vi "SO55 Initialize.vi"(1 "error in":errorcluster) -> (0 "error out":errorcluster, 2 "Settings Out":T1)   [LabVIEW 2012]
uses:
  SO55 Settings Cluster.ctl
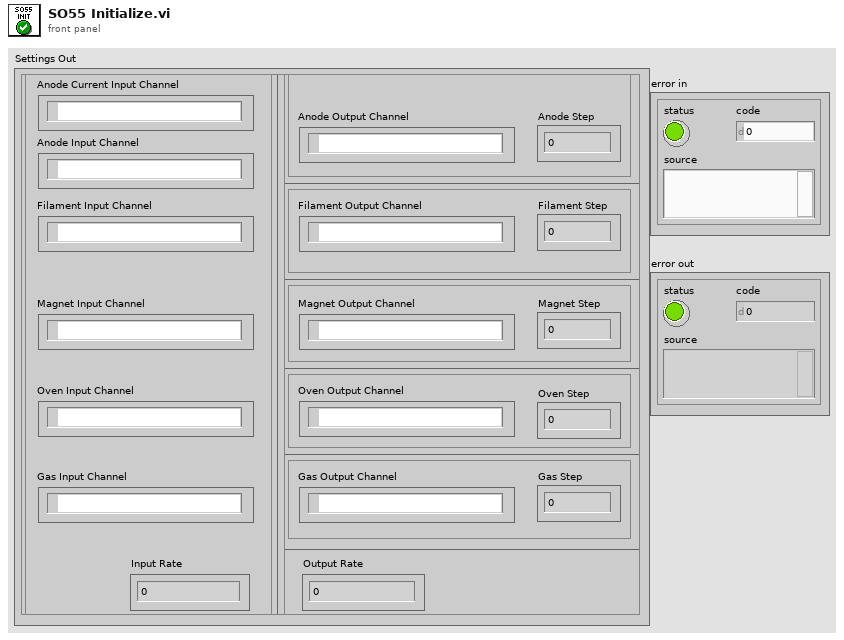
[diagram p1: front panel]
types:
  T1 = typedef "SO55 Settings Cluster.ctl" = cluster{"Input":cluster{"Anode Input Channel":tag, "Filament Input Channel":tag, "Magnet Input Channel":tag, "Oven Input Channel":tag, "Gas Input Channel":tag, "Input Rate":dbl, "Anode Current Input Channel":tag}, "Output":cluster{"Anode":cluster{"Anode Output Channel":tag, "Anode Step":dbl}, "Filament":cluster{"Filament Output Channel":tag, "Filament Step":dbl}, "Magnet":cluster{"Magnet Output Channel":tag, "Magnet Step":dbl}, "Oven":cluster{"Oven Output Channel":tag, "Oven Step":dbl}, "Gas":cluster{"Gas Output Channel":tag, "Gas Step":dbl}, "Output Rate":dbl}}
  T2 = enum16{"open", "replace", "create", "open or create", "replace or create", "replace or create with confirmation"}
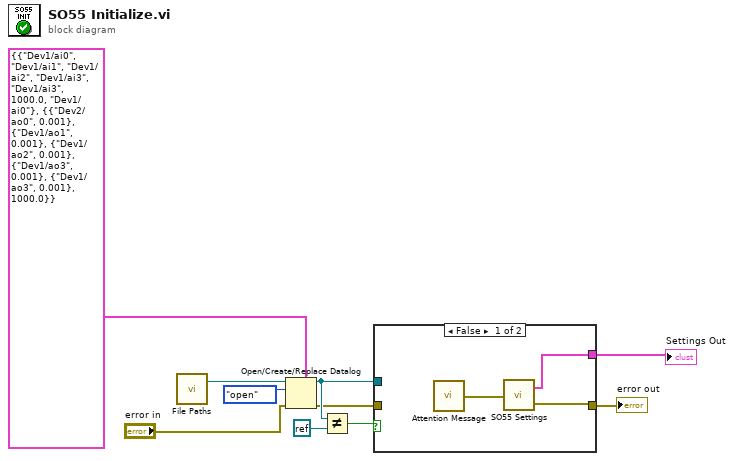
[diagram p0: block diagram]
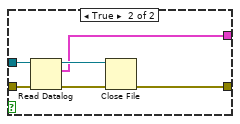
[diagram p2: hidden frame]
diagram:
  n1 = call "File Paths.vi"() -> ("SO55 Settings path"=w10:path)  [unwired: 1 out]
  n2 = Open/Create/Replace Datalog(5:T1 {"Input"={"Anode Input Channel"="Dev1/ai0", "Filament Input Channel"="Dev1/ai1", "Magnet Input Channel"="Dev1/ai2", "Oven Input Channel"="Dev1/ai3", "Gas Input Channel"="Dev1/ai3", "Input Rate"=1000.0, "Anode Current Input Channel"="Dev1/ai0"}, "Output"={"Anode"={"Anode Output Channel"="Dev2/ao0", "Anode Step"=0.001}, "Filament"={"Filament Output Channel"="Dev1/ao1", "Filament Step"=0.001}, "Magnet"={"Magnet Output Channel"="Dev1/ao2", "Magnet Step"=0.001}, "Oven"={"Oven Output Channel"="Dev1/ao3", "Oven Step"=0.001}, "Gas"={"Gas Output Channel"="Dev1/ao3", "Gas Step"=0.001}, "Output Rate"=1000.0}}, 8:"error in", 10:T2."open" ("operation (0:open)"), 11:w10) -> (0:w6:errorcluster, 3:w7:refnum<k1>)  [unwired: 2 in, 1 out]
  n3 = Not Equal?(x=w7, y=refnum<k0> refnum) -> (x != y?=w5:bool)
  n4 = case shown="False" w5 {
    tunnel: w6 -> [_ w16]
    tunnel: w7 -> [_ w17]
    tunnel: [w11 w15] -> w1
    tunnel: [w12 w14] -> w9
    frame False {
      n5 = call "Attention Message.vi"() -> ("Error Out"=w13:errorcluster)  [unwired: 1 in]
      n6 = call "SO55 Settings.vi"("Error In"=w13) -> ("Settings Out"=w11:T1, "Error Out"=w12:errorcluster)
    }
    frame True {
      n7 = Read Datalog(4:w16, 7:w17) -> (0:w19:errorcluster, 2:w15:T1, 3:w18:refnum<k1>)  [unwired: 1 in]
      n8 = Close File(refnum=w18, error in=w19) -> (error out=w14:errorcluster)  [unwired: 1 out]
    }
  }
  "error out" <- w9
  "Settings Out" <- w1
